vi "EXAMPLE_MULTITHREAD.vi"() -> ()   [LabVIEW 2017]
uses:
  a657961d-6c69-443e-8a94-87e847e8afca.vi
  46a5d0b1-31a7-4634-b485-2dd57def936d.vi
  d2a29e7f-7a10-4ef4-95c2-af8e2a57b835.vi
  fda3db9f-a2b2-414c-9bd7-69cd5009c9b8.vi
  TagDB/_Support/DataAccess/_NameCacher.vi
  TagDB/_Support/DataAccess/_datatypeChecker.vi
  TagDB/_Support/DataAccess/TagDB Ref to DVR.vi
  <vilib>/Utility/Data Type/Get Type Information.vi
  <vilib>/Utility/error.llb/Trim Whitespace.vi
  TagDB/_Support/Error/_[error50000]Invalid DB REF.vi
  TagDB/_Support/Error/_[error50002]Invalid DataType.vi
  TagDB/TagDB(DEV).lvlib
panel:
  in  "stop":bool
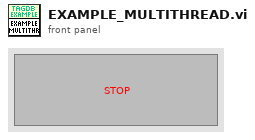
[diagram p1: front panel]
types:
  T1 = cluster{"number":i32, "boolean":bool, "abcdef":cluster{"number":i32, "boolean":bool}}
  T2 = typedef "TagDB(DEV).lvlib/TagContainer.ctl" = refnum<k1>
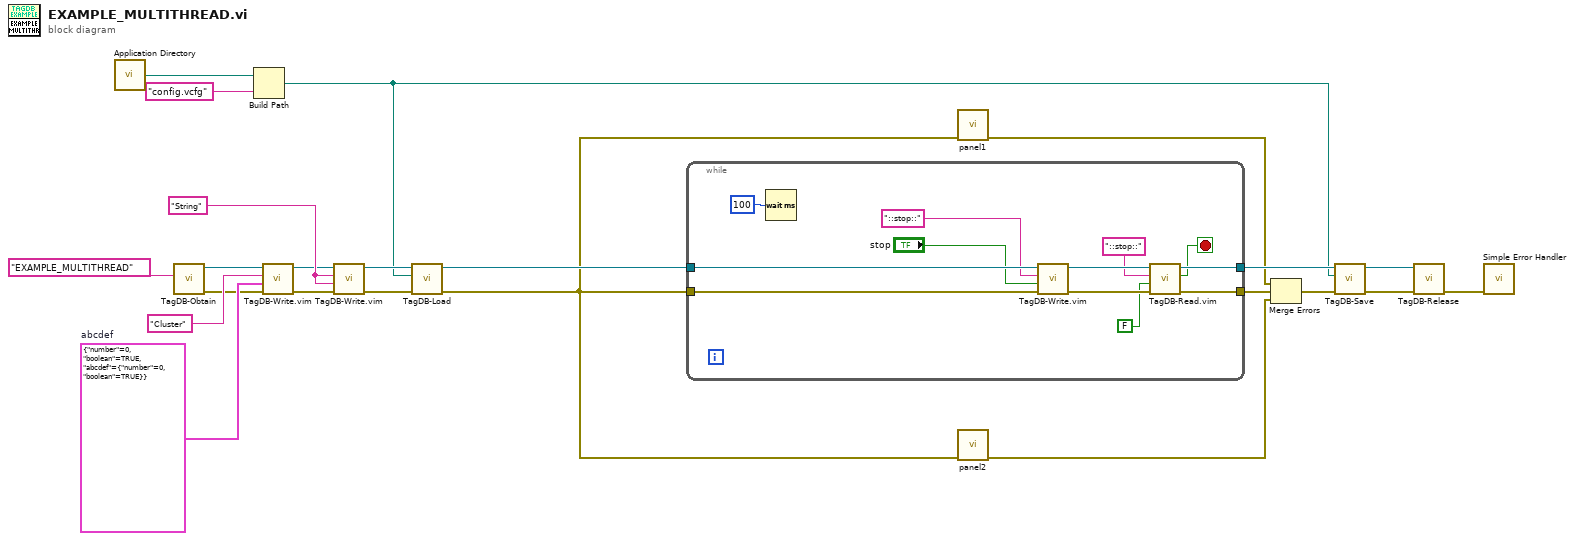
[diagram p0: block diagram]
diagram:
  w8 = T1 {"number"=0, "boolean"=TRUE, "abcdef"={"number"=0, "boolean"=TRUE}}  # abcdef
  w14 = "String" ("String")
  n1 = call <vilib>:"Application Directory.vi"() -> ("Application Directory"=w20:path)
  n2 = call "TagDB-Obtain.vi"("name (unnamed)"="EXAMPLE_MULTITHREAD") -> ("error out"=w3:errorcluster, "TagContainer"=w4:T2)  [unwired: 4 in, 1 out]
  n3 = Build Path(base path=w20, name or relative path="config.vcfg") -> (appended path=w5:path)
  n4 = call "TagDB-Write.vim"("error in (no error)"=w3, "Value"=w8, "name"="Cluster", "TagContainer"=w4) -> ("error out"=w10:errorcluster, "TagContainer(dup)"=w11:T2)  [unwired: 5 in, 1 out]
  n5 = call "TagDB-Write.vim"("error in (no error)"=w10, "Value"=w14, "name"=w14, "TagContainer"=w11) -> ("error out"=w15:errorcluster, "TagContainer(dup)"=w16:T2)  [unwired: 5 in, 1 out]
  n6 = call "TagDB-Load.vi"("error in (no error)"=w15, "file path(empty for default)"=w5, "DB Ref"=w16) -> ("error out"=w12:errorcluster, "DB Ref(dup)"=w13:T2)  [unwired: 7 in]
  n7 = while {
    tunnel: w13 -> [w33]
    tunnel: w12 -> [w34]
    tunnel: [w26] -> w23
    tunnel: [w29] -> w18
    stop <- w25 stop-if-true
    n8 = Wait (ms)(milliseconds to wait=u32 100) -> ()  [unwired: 1 out]
    n9 = call "TagDB-Write.vim"("error in (no error)"=w34, "Value"="stop", "name"="::stop::", "TagContainer"=w33) -> ("error out"=w27:errorcluster, "TagContainer(dup)"=w30:T2)  [unwired: 5 in, 1 out]
    n10 = call "TagDB-Read.vim"("error in (no error)"=w27, "Type"=FALSE, "name"="::stop::", "TagContainer"=w30) -> ("error out"=w26:errorcluster, "Value"=w25:bool, "TagContainer(dup)"=w29:T2)  [unwired: 2 in, 3 out]
  }
  n11 = call "panel1.vi"("error in (no error)"=w12) -> ("error out"=w2:errorcluster)  [unwired: 10 in]
  n12 = call "panel2.vi"("error in (no error)"=w12) -> ("error out"=w21:errorcluster)  [unwired: 10 in]
  n13 = Merge Errors(w2, w23, w21) -> (w17:errorcluster)
  n14 = call "TagDB-Save.vi"("error in (no error)"=w17, "file path(empty for default)"=w5, "DB Ref"=w18) -> ("error out"=w6:errorcluster, "DB Ref(dup)"=w7:T2)  [unwired: 7 in]
  n15 = call "TagDB-Release.vi"("error in (no error)"=w6, "TagContainer"=w7) -> ("error out"=w22:errorcluster)  [unwired: 9 in]
  n16 = call <vilib>:"Simple Error Handler.vi"("error in (no error)"=w22) -> ()  [unwired: 4 in, 5 out]
